vi "calibrate.vi"() -> (3 "function return":i32)   [LabVIEW 2017, in "Calibration.lvlib"]
doc: "extern \"C\" __declspec(dllexport) int calibrate(int argc, char* argv[]);\n\nextern \"C\" __declspec(dllexport) int calibrate();"
uses:
  <userlib>/HapticSTM/Feedbackless - Testdata/Project/feedbackless.lvproj/Proj/Feedbackless Folder/Calibration/Calibration.lvlib
  <userlib>/Calibration/Calibration.dll
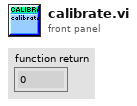
[diagram p1: front panel]
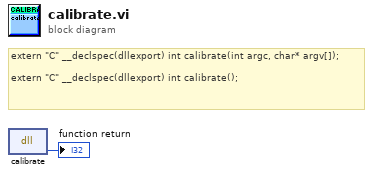
[diagram p0: block diagram]
diagram:
  # "extern \"C\" __declspec(dllexport) int calibrate(int argc, char* argv[]);\n\nextern \"C\" __declspec(dllexport) int calibrate();"
  n1 = dll-call lib="C:/Program Files/National Instruments/LabVIEW 2019/user.lib/Calibration/Calibration.*" fn="calibrate"() -> (→"function return":i32)  [unwired: 3 in, 2 out]
